vi "set datatype.vi"(8 "error in (no error)":errorcluster, 10 "datatype":T1, 11 "JSON Helper in":refnum<class "JSON Helper.lvclass">) -> (0 "error out":errorcluster, 3 "JSON Helper out":refnum<class "JSON Helper.lvclass">)   [LabVIEW 2016, in "JSON Helper.lvclass"]
uses:
  JSON Helper.lvclass
  JSON Types.ctl
  JSON Helper.lvclass/JSON Helper.ctl
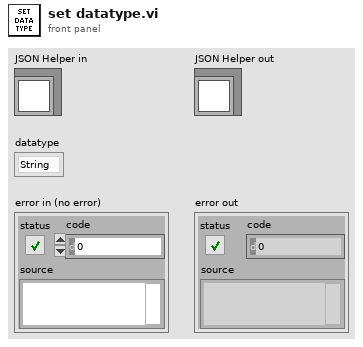
[diagram p1: front panel]
types:
  T1 = typedef "JSON Helper.lvclass/JSON Types.ctl" = enum16{"String", "Numeric", "Boolean", "NULL", "Object", "Array"}
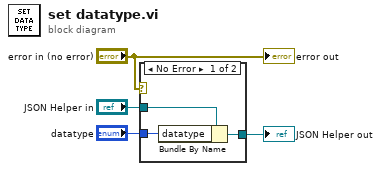
[diagram p0: block diagram]
diagram:
  n1 = case shown="No Error" "error in (no error)" {
    tunnel: "datatype" -> [w7 _]
    tunnel: [w6 w8] -> w3
    tunnel: "JSON Helper in" -> [w5 w8]
    frame No Error {
      n2 = Bundle By Name(cluster=w5, "datatype"=w7) -> (w6:refnum<class "JSON Helper.lvclass">)
    }
    frame Error {
    }
  }
  "JSON Helper out" <- w3
  "error out" <- "error in (no error)"
